vi "Copy All.vi"(8 "error in (no error)":errorcluster, 10 "dst Pointer in":refnum<class "Pointer.lvclass">, 11 "src Pointer in":refnum<class "Pointer.lvclass">) -> (0 "error out":errorcluster, 2 "dst Pointer out":refnum<class "Pointer.lvclass">, 3 "src Pointer out":refnum<class "Pointer.lvclass">)   [LabVIEW 2020, in "Memory Manager.lvlib" / "Pointer.lvclass"]
doc: "Copies all bytes specified by <b>src Pointer</b> to <b>dst Pointer</b>."
uses:
  Pointer.lvclass
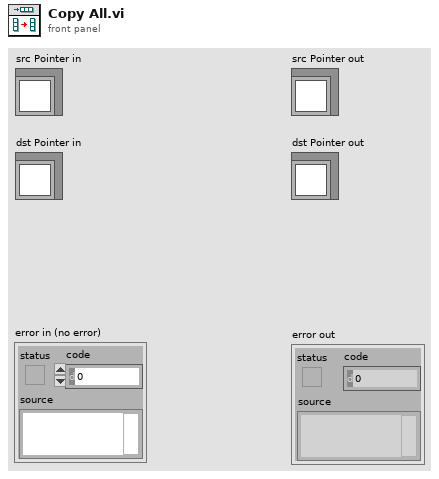
[diagram p1: front panel]
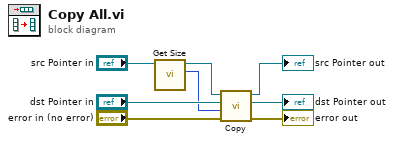
[diagram p0: block diagram]
diagram:
  n1 = call "Get Size.vi"("Pointer in"="src Pointer in") -> ("size"=w5:u64, "Pointer out"=w7:refnum<class "Pointer.lvclass">)  [unwired: 9 in]
  n2 = call "Copy.vi"("error in (no error)"="error in (no error)", "size"=w5, "dst Pointer in"="dst Pointer in", "src Pointer in"=w7) -> ("error out"=→"error out":errorcluster, "dst Pointer out"=→"dst Pointer out":refnum<class "Pointer.lvclass">, "src Pointer out"=→"src Pointer out":refnum<class "Pointer.lvclass">)  [unwired: 4 in, 1 out]
